vi "DVRtoRef.vi"(10 "DVR":refnum<data-value>) -> (2 "Ref":u32)   [LabVIEW 2019, in "RemoteControl.ZMQ.lvlib" / "ZMQ.ContextManager.lvlib"]
uses:
  ZMQ.ContextManager.lvlib
  Typedefs/Context--Cluster.ctl
  <vilib>/addons/zeromq/zmq_context.lvclass
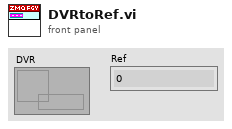
[diagram p1: front panel]
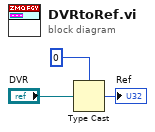
[diagram p0: block diagram]
diagram:
  n1 = Type Cast(type=u32 0 ("Ref"), x="DVR") -> (*(type *) &x=→"Ref":u32)
